vi "LoopScript_ChangeSpeed.vi"() -> ()   [LabVIEW 2017]
uses:
  AODControl/AODGlobals.vi
  ImageAcquisitionProgram/ImageAcquisitionLibrary/GlobalFrontPanelReferences.vi
  AODControl/AODControl.lvlib
  ImageAcquisitionProgram/ImageAcquisitionLibrary/ImageAcquisitionLibrary.lvlib
panel:
  out "iteration":i32
  out "initial rotation speed":dbl
  in  "waiting time (s)":i32
  out "current speed":dbl
  in  "Final speed":dbl format="%#_13g"
  in  "N points":i32
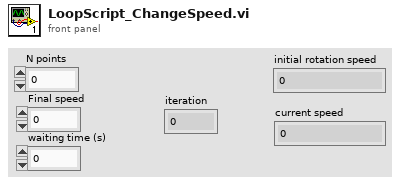
[diagram p1: front panel]
types:
  T1 = typedef "AODControl.lvlib/InterfaceReferences.ctl" = cluster{"AOD Points Display":refnum<vi>, "AOD Array":refnum<vi>, "AOD Array Size":refnum<vi>, "Replace Array List":refnum<vi>, "Replace List":refnum<vi>, "Remove":refnum<vi>, "Index":refnum<vi>, "Move":refnum<vi>, "X":refnum<vi>, "Y":refnum<vi>, "Add":refnum<vi>, "Load":refnum<vi>, "Save":refnum<vi>, "Exit":refnum<vi>, "Dynamic":refnum<vi>, "Rotate":refnum<vi>, "Rotation Speed":refnum<vi>, "Scaling Speed":refnum<vi>, "X Trans Speed":refnum<vi>, "Y Trans Speed":refnum<vi>, "Movie Array":refnum<vi>}
  T2 = typedef "ImageAcquisitionLibrary.lvlib/References.ctl" = cluster{"Acquire":refnum<vi>, "Rec":refnum<vi>, "Tracking":refnum<vi>, "Settings":refnum<vi>, "Stop":refnum<vi>, "Initialized?":bool, "ImDisplay":refnum<vi>}
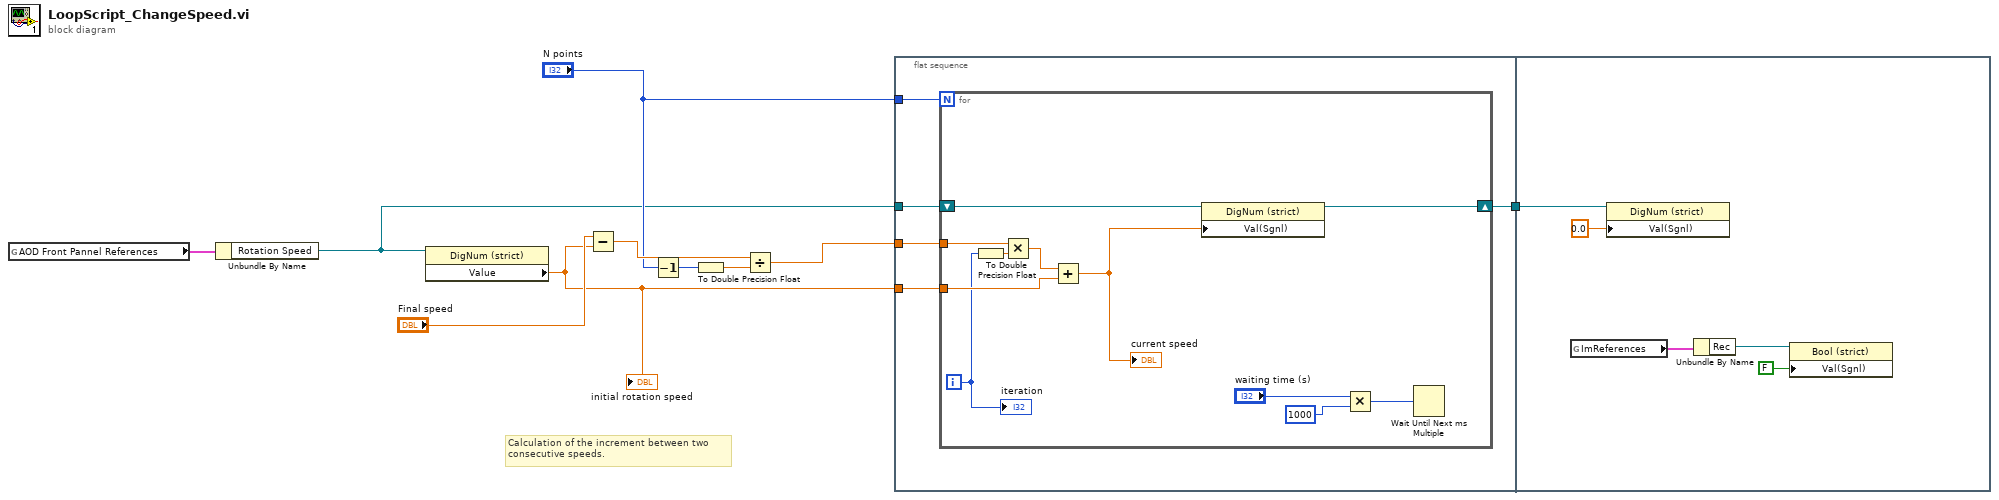
[diagram p0: block diagram]
diagram:
  # "Calculation of the increment between two\nconsecutive speeds."
  n1 = global read "AODGlobals.vi" "AOD Front Pannel References"() -> (w6:T1)
  n2 = Unbundle By Name(w6) -> ("Rotation Speed"=w4:refnum<vi>)
  n3 = property class="DigNum (strict)"(reference=w4) -> ("Value"=w3:dbl)  [unwired: 1 in, 2 out]
  "initial rotation speed" <- w3
  n4 = Subtract(x="Final speed", y=w3) -> (x-y=w9:dbl)
  n5 = Decrement(x="N points") -> (x-1=w1:i32)
  n6 = To Double Precision Float(number=w1) -> (double precision float=w8:dbl)
  n7 = Divide(x=w9, y=w8) -> (x/y=w7:dbl)
  n8 = flat-sequence {
    tunnel: w7 -> [w15]
    tunnel: "N points" -> [w14]
    tunnel: w4 -> [w13]
    tunnel: w3 -> [w12]
    tunnel: [w11] -> w2
    tunnel: w2 -> [w28]
    frame #0 {
      n9 = for {
        N: w14 -> [_]
        tunnel: w15 -> [w26]
        tunnel: w12 -> [w24]
        shift-right: [w19] -> w11
        shift-left: w13 -> [w20]
        i -> [w16]
        n10 = To Double Precision Float(number=w16) -> (double precision float=w25:dbl)
        n11 = Multiply(x=w26, y=w25) -> (x*y=w23:dbl)
        n12 = Add(x=w23, y=w24) -> (x+y=w18:dbl)
        "current speed" <- w18
        n13 = property class="DigNum (strict)"(reference=w20, "Val(Sgnl)"=w18) -> (reference out=w19:refnum<vi>)  [unwired: 1 in, 1 out]
        n14 = Multiply(x="waiting time (s)", y=1000) -> (x*y=w17:i32)
        n15 = Wait Until Next ms Multiple(millisecond multiple=w17) -> ()  [unwired: 1 out]
        "iteration" <- w16
      }
    }
    frame #1 {
      n16 = global read "GlobalFrontPanelReferences.vi" "ImReferences"() -> (w30:T2)
      n17 = property class="DigNum (strict)"(reference=w28, "Val(Sgnl)"=0.0) -> ()  [unwired: 1 in, 2 out]
      n18 = Unbundle By Name(w30) -> ("Rec"=w31:refnum<vi>)
      n19 = property class="Bool (strict)"(reference=w31, "Val(Sgnl)"=FALSE) -> ()  [unwired: 1 in, 2 out]
    }
  }
